vi "Select System By Name.vi"(8 "error in (no error)":errorcluster, 10 "SystemlName":string, 11 "SystemsIn":refnum<class "BME_DG_System.lvclass">[](array[class])) -> (0 "error out":errorcluster, 2 "BME_DG_System out":refnum<class "BME_DG_System.lvclass">, 3 "SystemsOut":refnum<class "BME_DG_System.lvclass">[](array[class]))   [LabVIEW 2009, in "POLARIS BME DG.lvlib" / "BME_DG_System.lvclass"]
uses:
  BME_DG_System.lvclass
  BME_DG_System.lvclass/BME_DG_System.ctl
  POLARIS BME DG.lvlib
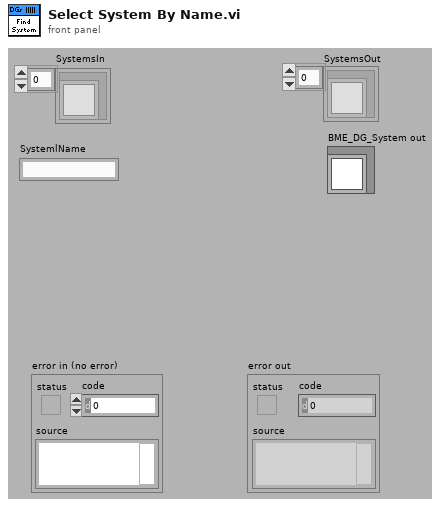
[diagram p1: front panel]
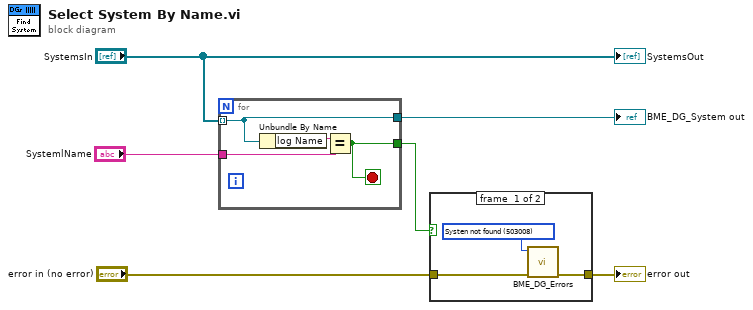
[diagram p0: block diagram]
diagram:
  n1 = for {
    tunnel: "SystemsIn" -> [w8] mode=indexing
    tunnel: "SystemlName" -> [w9]
    tunnel: [w8] -> w4
    tunnel: [w7] -> w3
    stop <- w7 stop-if-true
    n2 = Unbundle By Name(w8) -> ("log Name"=w10:string)
    n3 = Equal?(x=w10, y=w9) -> (x = y?=w7:bool)
  }
  "BME_DG_System out" <- w4
  n4 = case shown="False" w3 {
    tunnel: "error in (no error)" -> [w13 w14]
    tunnel: [w12 w14] -> w1
    frame #0 {
      w11 = 503008 items=["Channel refers itself"=503001, "Deadloop"=503002, "Negative Delay"=503003, "Delay Card not found"=503004, "Channel not found"=503005, "Parse Error"=503006, "Not Supported"=503007, "Systen not found"=503008, "To much masters"=503009, "None master in Syterm"=503010, "InterruptError"=503011, "ChnlPeriodeWarning"=503012] ("error")
      n5 = call "BME_DG_Errors.vi"("error in (no error)"=w13, "error"=w11) -> ("error out"=w12:errorcluster)  [unwired: 9 in]
    }
    frame #1 {
    }
  }
  "error out" <- w1
  "SystemsOut" <- "SystemsIn"
